vi "ROS_Master_updateNode.vi"(0 "ROS_Master in":T1, 1 "PubSub":T2) -> (2 "ROS_Master out":T1, 3 "Shutdown URI":string, 4 "shutdown needed?":bool)   [LabVIEW 2015]
doc: "Updates node with master, registers new nodes with master, and checks whether or not nodes have same IP"
uses:
  ROS_Topic.ctl
  ROS_Master.ctl
  ROS_Node.ctl
  ROS_Service.ctl
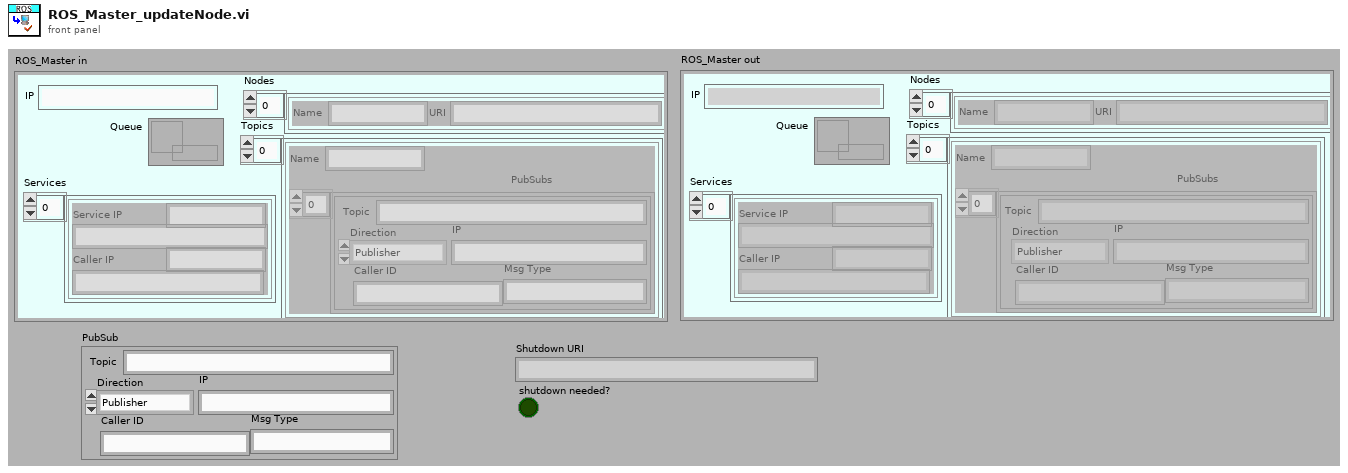
[diagram p1: front panel]
types:
  T1 = typedef "ROS_Master.ctl" = cluster{"IP":string, "Topics":cluster{"Name":string, "PubSubs":T2[]}[], "Nodes":T3[], "Services":T4[], "Queue":refnum<queue>}
  T2 = typedef "ROS_Topic.ctl" = cluster{"Caller ID":string, "IP":string, "Msg Type":string, "Direction":enum16{"Publisher", "Subscriber"}, "Topic":string}
  T3 = typedef "ROS_Node.ctl" = cluster{"Name":string, "URI":string}
  T4 = typedef "ROS_Service.ctl" = cluster{"Service":string, "Service IP":string, "Caller IP":string, "Caller ID":string}
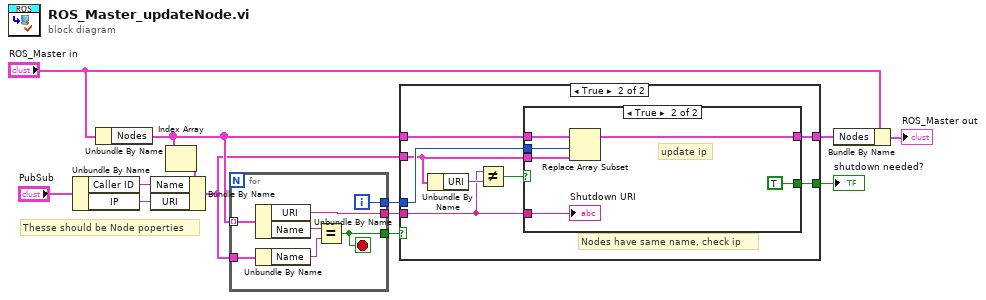
[diagram p0: block diagram]
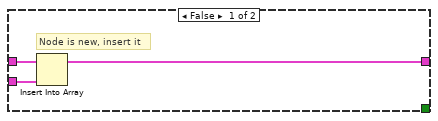
[diagram p2: hidden frame]
diagram:
  # "Thesse should be Node poperties"
  n1 = Unbundle By Name("PubSub") -> ("Caller ID"=w6:string, "IP"=w5:string)
  n2 = Unbundle By Name("ROS_Master in") -> ("Nodes"=w3:T3[])
  n3 = Index Array(array=w3) -> (element=w2:T3)  [unwired: 1 in]
  n4 = Bundle By Name(cluster=w2, "Name"=w6, "URI"=w5) -> (w1:T3)
  n5 = for {
    tunnel: w1 -> [w19]
    tunnel: w3 -> [w20] mode=indexing
    tunnel: [w16] -> w13
    tunnel: [w15] -> w12
    tunnel: [w14] -> w11
    i -> [w14]
    stop <- w16 stop-if-true
    n6 = Unbundle By Name(w20) -> ("URI"=w15:string, "Name"=w18:string)
    n7 = Unbundle By Name(w19) -> ("Name"=w17:string)
    n8 = Equal?(x=w18, y=w17) -> (x = y?=w16:bool)
  }
  n9 = case shown="True" w13 {
    tunnel: w12 -> [_ w24]
    tunnel: w1 -> [w22 w27]
    tunnel: w3 -> [w23 w29]
    tunnel: w11 -> [_ w28]
    tunnel: [_ w30] -> w10
    tunnel: [w21 w25] -> w9
    frame False {
      # "Node is new, insert it"
      n10 = Insert Into Array(array=w23, new element=w22) -> (w21:T3[])  [unwired: 1 in]
    }
    frame True {
      # "Nodes have same name, check ip"
      n11 = Unbundle By Name(w27) -> ("URI"=w26:string)
      n12 = Not Equal?(x=w24, y=w26) -> (x != y?=w31:bool)
      n13 = case shown="True" w31 {
        tunnel: [_ TRUE] -> w30
        tunnel: w29 -> [w32 w37]
        tunnel: w28 -> [_ w36]
        tunnel: w27 -> [_ w35]
        tunnel: [w32 w34] -> w25
        tunnel: w24 -> [_ w33]
        frame False {
        }
        frame True {
          # "update ip"
          n14 = Replace Array Subset(array=w37, new element=w35, index=w36) -> (w34:T3[])
          "Shutdown URI" <- w33
        }
      }
    }
  }
  "shutdown needed?" <- w10
  n15 = Bundle By Name(cluster="ROS_Master in", "Nodes"=w9) -> (→"ROS_Master out":T1)
